vi "FestoCPX.Station.Prod.Unload.vi"(8 "error in":errorcluster, 9 "retries (0)":i32, 10 "SuckerID":i32, 11 "Slot":T1) -> (0 "error out":errorcluster)   [LabVIEW 2016]
uses:
  Station/Station.ProductSlot.ctl
  tools/Translator/Translator.Message.ctl
  tools/EventLog/EventLog.EventSource.ctl
  Station/Station.ValvePosition.ctl
  tools/EventLog/EventLog.CreateError(single).vi
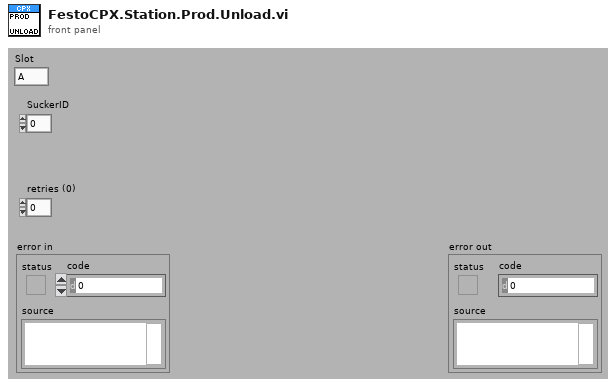
[diagram p1: front panel]
types:
  T1 = typedef "Station.ProductSlot.ctl" = enum8{"A", "B"}
  T2 = typedef "Translator.Message.ctl" = enum16{"-", "Event confirmed", "Log out", "Log in", "Shutdown", "Cancel", "Start", "Begin time", "End time", "Duration", "Service Mode", "Ignore Results", "On", "Off", "OK", "NOK", "NOK %s", "Home", "Work", "Close", "Open", "In progress...", "Missing", "Empty", "Hardware failure", "Initial", "Default", "Total", "Out of range", "Error %d >> %s", "Error %d >> %s >> %s", "Msg %d >> %s", "Laser msg %d %s", "Laser cmd error %s %d", "Laser cmd failed %s", "Laser cmd warning %s", "Laser disconnected", "Laser status %s", "Laser already started", "Laser job unkonwn %s", "Laser job missing %s", "Laser job select failure %s", "Unable to start laser printing (%s)", "Unable to stop laser printing (%s)", "Laser marking aborted", "Laser marking timeout", "Unable to reset Laser Interlock (%s)", "Unable to trigger Laser. Laser not ready (%s)", "Laser job '%s' coordinates not configured", "Starting %s", "Quitting %s", "Configured", "Initializing", "Quitting", "Loading", "Running", "Stopped", "Summary", "Laser", "Do you want to continue?", "Do you want to delete the configuration?", "The configuration is being used by an order. Unable to delete!", "Press confirm button", "Station is not based. Do you want to exit?", "Station requires changeover. Do you want to run the test?", "Test options are not set as default. Do you want to continue?", "Product not detected. Do you want to continue?", "Product scan failed. Do you want to continue?", "Calibration", "Log out?", "System", "All", "IDLE", "Translating...%s", "Not found", "Alarm %s", "Run", "Skip", "Abort", "Repeat", "Please wait...", "Database disconnected", "Database disconnected - changeover disabled!", "Login to database successful", "Login to database failed: %d; %s", "Unable to check the product status of reference %d - database disconnected", "Unable to set the product status of reference %d - database disconnected", "Variant file backup %s", "Read steps (%s)", "Result", "Station armed!", "Station requires changeover!", "Select reference number...", "EMERGENCY BUTTON - press Control button", "EMERGENCY DOOR - press Control button", "Resetting Emergency...", "Unable to reset safety circuit - Emergency Button pressed", "Unable to reset safety circuit - Emergency Side Door open", "Station not based", "Station based", "Station not empty", "Station basing...", "No order", "Press Start to begin new order", "Scanning new order", "Order NOK. Correct or scan again", "Order OK. Press Accept", "Order ready", "Revolver incorrect", "Fork incorrect", "Revolver missing", "Revolver empty", "Container missing", "Offline results", "Offline statistics", "DMC Configurator", "Door open", "Close the front door", "Press start button", "Done. Open the front door", "Running...", "Running...%.1f %%", "Pause", "Pause. NOK container missing", "Pause. OK container missing", "Pause. Revolver empty", "Pause. Revolver missing", "Pause. Revolver incorrect", "Pause. Fork missing", "Pause. Fork incorrect", "Pause. Too many failures", "Pause. One slot is not working", "Pause. Unable to move product to slot", "Pause. Unable to move back product pusher", "Pause. Unable to lift product", "Pause. Unable to move back product lifter", "Pause. Unable to move product arm to Work", "Pause. Unable to move product arm to NOK", "Pause. Unable to move product arm to OK", "Pause. Unable to unsuck the NOK product", "Pause. Unable to drop the NOK product", "Pause. Product OK missing", "Pause. Unable to unsuck the OK product", "Pause. Unable to drop the OK product", "Stopping...", "File '%s' is missing", "File '%s' is broken", "File '%s' is running", "Log file started (%s)", "Log file ended (%s)", "Log file ignored (%s)", "Log file exported (%s)", "Log file export failed (%s)", "Wrong serial number in log file", "Wrong reference number in log file", "Test steps are missing", "%s = %.3f", "Process param '%s' not found in DB", "Process param '%s' wrong order", "Process param '%s' value %.3f out of limits (%.3f; %.3f)", "Step%d param '%s' not found in DB", "Step%d param '%s' wrong order", "Step%d param '%s' value %.3f out of limits (%.3f; %.3f)", "Step%d EV '%s' not found in DB", "Step%d EV '%s' wrong order", "\"%s\" not found in DB", "\"%s\" wrong order", "\"%s\" value %.3f out of limits (%.3f; %.3f)", "\"%s\" not found in software", "Process init (%s)", "Process started", "Process restarted", "Process run", "Process done", "Process aborted", "Process aborted at work", "Process aborted at home", "Process error", "Process error at home", "Process error at work", "Process close", "Select plate from the order to process", "Do you want to start the process?", "Do you want to repeat the process?", "There is unfinished order. Do you want to put the new order?", "Product %s %d OK", "Product %s %d NOK", "Unable to unload the slot %s. Product missing in the slot", "Unable to unload the slot %s. Product already in the arm", "Unable to accept the product as OK. Product missing in slot %s", "Unable to accept the product as OK. Product could not drop into the container at slot %s", "Unable to accept the product as NOK. Product could not drop into the container at slot %s", "Scan failed. Error %s", "Scan failed. Scanner disconnected", "Scan failed. Wrong Wabco number %d, limit (%d,%d)", "Scan failed. Wrong serial number %d, limit (%d,%d)", "Scan failed. Wrong date %d, limit (%d,%d)", "Scan failed. Wrong product wabco number %d (expected %d)", "Scan failed. Wrong product serial number %d (expected > 0)", "Scan OK %s", "Scan failed. Unable to determine table position (%s)", "Scan failed. Timeout", "Tune failed. Scanner disconnected", "Tune failed. Timeout", "%s = %d", "%s = %d->%d", "Unable to set %s = %.2f - Air Pressure Inside off", "Unable to set digital output '%s' = %d", "Unable to activate air pressure inside - timeout", "Unable to activate air pressure inside - aborted", "Unable to switch on Air Main Valve - Air Pressure Inlet off", "Unable to switch on Air Main Valve - Door open", "Unable to switch off Air Main Valve - timeout", "Unable to switch off Air Main Valve - aborted", "Unable to rotate Table - timeout", "Unable to rotate Table - aborted", "Unable to rotate Table - Product Move not in Home position", "Unable to rotate Table - Air Pressure Inside off", "Unable to rotate Table - Product Lift A not in Home position", "Unable to rotate Table - Product Lift B not in Home position", "Unable to rotate Table - unlock before movement timeout", "Unable to rotate Table - lock after movement timeout", "Unable to move Table Lock to %s position - timeout", "Unable to move Table Lock to %s position - aborted", "Unable to move Table Lock to %s position - Air Pressure Inside off", "Unable to move Table Lock to %s position - Table not in position", "Unable to move Product Lift A to %s position - timeout", "Unable to move Product Lift B to %s position - timeout", "Unable to move Product Lift A to %s position - aborted", "Unable to move Product Lift B to %s position - aborted", "Unable to move Product Lift A to %s position - Air Pressure Inside off", "Unable to move Product Lift B to %s position - Air Pressure Inside off", "Unable to move Product Lift A to %s position - Table not locked", "Unable to move Product Lift B to %s position - Table not locked", "Unable to move Product Lift A to %s position - Product Arm not in Work position", "Unable to move Product Lift B to %s position - Product Arm not in Work position", "Unable to set Product Suction Gripper %s to %s - timeout", "Unable to set Product Suction Gripper %s to %s - aborted", "Unable to set Product Suction Gripper %s to %s - Air Pressure Inside off", "Unable to set Product Suction Gripper %s to %s - Table slot unkown", "Unable to move Product Arm to %s position - timeout", "Unable to move Product Arm to %s position - aborted", "Unable to move Product Arm to %s position - Air Pressure Inside off", "Unable to move Product Arm to %s position - Product Lift A not in Home position", "Unable to move Product Arm to %s position - Product Lift B not in Home position", "Unable to move Product to %s position - timeout", "Unable to move Product to %s position - aborted", "Unable to move Product to %s position - Air Pressure Inside off", "Unable to move Product to %s position - Table not in position"}
  T3 = typedef "Station.ValvePosition.ctl" = enum16{"Home", "Work"}
  T4 = typedef "EventLog.EventSource.ctl" = enum16{"All", "Gui", "Ref", "File", "Arch", "Seq", "CPX", "Proda", "Laser", "Scan.P", "Scan.O"}
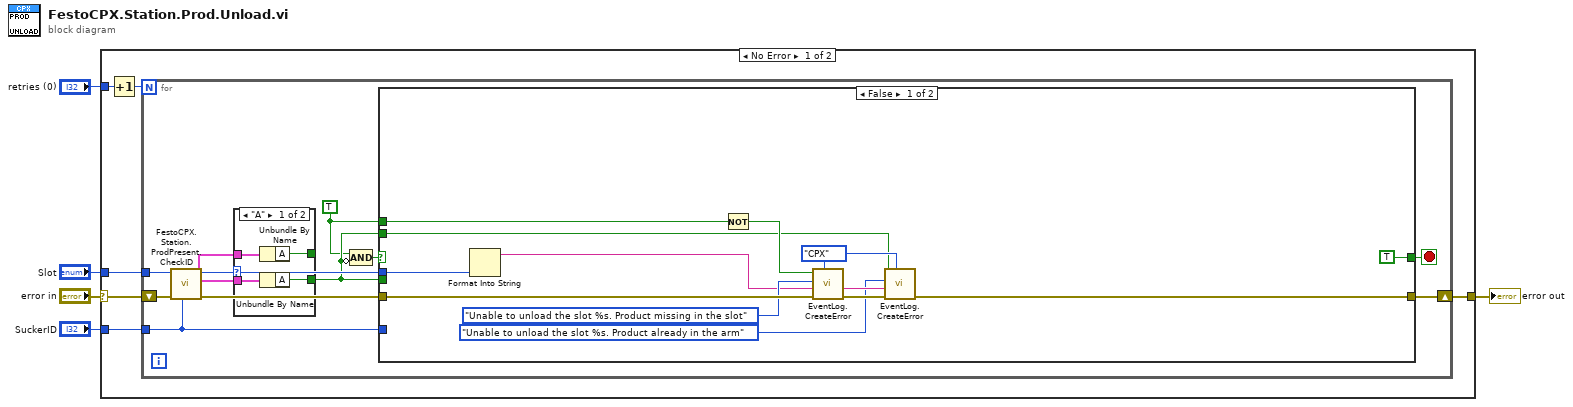
[diagram p0: block diagram]
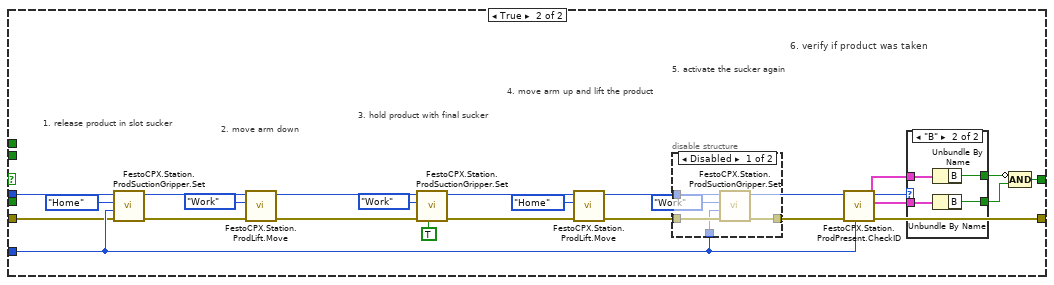
[diagram p2: hidden frame]
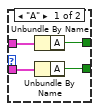
[diagram p4: hidden frame]
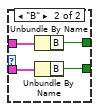
[diagram p5: hidden frame]
diagram:
  n1 = case shown="No Error" "error in" {
    selector: "error in" -> [w6 w76]
    tunnel: [w11 w76] -> w5
    tunnel: "Slot" -> [w10 _]
    tunnel: "SuckerID" -> [w9 _]
    tunnel: "retries (0)" -> [w7 _]
    frame No Error {
      n2 = Increment(x=w7) -> (x+1=w8:i32)
      n3 = for {
        N: w8 -> [_]
        tunnel: w10 -> [w20]
        tunnel: w9 -> [w17]
        shift-right: [w22] -> w11
        shift-left: w6 -> [w19]
        stop <- w15 stop-if-true
        w12 = TRUE ("value")
        n4 = call "FestoCPX.Station.ProdPresent.CheckID.vi"("SuckerID (0: Final)"=w17, "error in"=w19) -> ("error out"=w18:errorcluster, "Present.Final"=w21:cluster{"A":bool, "B":bool}, "Present.SuckerID"=w16:cluster{"A":bool, "B":bool})  [unwired: 6 in, 1 out]
        n5 = case shown="\"A\"" w20 {
          tunnel: w21 -> [w71 w75]
          tunnel: w16 -> [w70 w74]
          tunnel: [w69 w73] -> _
          tunnel: [w68 w72] -> w13
          frame "A" {
            n6 = Unbundle By Name(w70) -> ("A"=w69:bool)
            n7 = Unbundle By Name(w71) -> ("A"=w68:bool)
          }
          frame "B" {
            n8 = Unbundle By Name(w74) -> ("B"=w73:bool)
            n9 = Unbundle By Name(w75) -> ("B"=w72:bool)
          }
        }
        n10 = Compound Arithmetic op=AND(w12, invert w13) -> (w14:bool)
        n11 = case shown="False" w14 {
          tunnel: [w29 w46] -> w22
          tunnel: w20 -> [w31 w41]
          tunnel: w18 -> [w34 w36]
          tunnel: w17 -> [_ w38]
          tunnel: [TRUE w42] -> w15
          tunnel: w13 -> [_ _]
          tunnel: w12 -> [w24 _]
          tunnel: w13 -> [w23 _]
          frame False {
            w28 = EventLog.EventSource."CPX" ("Source (All)")
            n12 = Format Into String(w31) -> (resulting string=w27:string)  [unwired: 3 in, 1 out]
            n13 = Not(x=w24) -> (.not. x?=w25:bool)
            n14 = call-poly "EventLog.CreateError.vi"("Source (All)"=w28, "error in"=w34, "arg"=w27, "msg"=Translator.Message."Unable to unload the slot %s. Product missing in the slot", "create (T)"=w25) -> ("error out"=w30:errorcluster)  [unwired: 6 in]
            n15 = call-poly "EventLog.CreateError.vi"("Source (All)"=w28, "error in"=w30, "arg"=w27, "msg"=Translator.Message."Unable to unload the slot %s. Product already in the arm", "create (T)"=w23) -> ("error out"=w29:errorcluster)  [unwired: 6 in]
          }
          frame True {
            # "5. activate the sucker again"
            # "2. move arm down"
            # "6. verify if product was taken"
            # "4. move arm up and lift the product"
            # "3. hold product with final sucker"
            # "1. release product in slot sucker"
            n16 = call "FestoCPX.Station.ProdSuctionGripper.Set.vi"("error in"=w36, "Sucker (0: Final)"=w38, "Position"=Station.ValvePosition."Home", "Slot"=w41) -> ("error out"=w35:errorcluster)  [unwired: 6 in, 1 out]
            n17 = call "FestoCPX.Station.ProdLift.Move.vi"("error in"=w35, "Position"=Station.ValvePosition."Work", "Slot"=w41) -> ("error out"=w37:errorcluster)  [unwired: 8 in]
            n18 = call "FestoCPX.Station.ProdSuctionGripper.Set.vi"("wait for product (F)"=TRUE, "error in"=w37, "Position"=Station.ValvePosition."Work", "Slot"=w41) -> ("error out"=w51:errorcluster)  [unwired: 6 in, 1 out]
            n19 = call "FestoCPX.Station.ProdLift.Move.vi"("error in"=w51, "Position"=Station.ValvePosition."Home", "Slot"=w41) -> ("error out"=w40:errorcluster)  [unwired: 8 in]
            n20 = disable-structure shown="Disabled" {
              disable-tunnel: w41 -> [w57 _]
              disable-tunnel: w40 -> [w56 w59]
              disable-tunnel: [w55 w59] -> w39
              disable-tunnel: w38 -> [w54 _]
              frame Disabled {
                n21 = call "FestoCPX.Station.ProdSuctionGripper.Set.vi"("error in"=w56, "Sucker (0: Final)"=w54, "Position"=Station.ValvePosition."Work", "Slot"=w57) -> ("error out"=w55:errorcluster)  [unwired: 6 in, 1 out]
              }
              frame Enabled {
              }
            }
            n22 = call "FestoCPX.Station.ProdPresent.CheckID.vi"("SuckerID (0: Final)"=w38, "error in"=w39) -> ("error out"=w46:errorcluster, "Present.Final"=w47:cluster{"A":bool, "B":bool}, "Present.SuckerID"=w43:cluster{"A":bool, "B":bool})  [unwired: 6 in, 1 out]
            n23 = case shown="\"B\"" w41 {
              tunnel: w47 -> [w63 w67]
              tunnel: w43 -> [w62 w66]
              tunnel: [w61 w65] -> w45
              tunnel: [w60 w64] -> w44
              frame "A" {
                n24 = Unbundle By Name(w62) -> ("A"=w61:bool)
                n25 = Unbundle By Name(w63) -> ("A"=w60:bool)
              }
              frame "B" {
                n26 = Unbundle By Name(w66) -> ("B"=w65:bool)
                n27 = Unbundle By Name(w67) -> ("B"=w64:bool)
              }
            }
            n28 = Compound Arithmetic op=AND(invert w45, w44) -> (w42:bool)
          }
        }
      }
    }
    frame Error {
    }
  }
  "error out" <- w5
